vi "TitleBar.CreateBroadcasts.vi"(8 "error in (no error)":errorcluster) -> (0 "error out":errorcluster, 3 "Broadcasts":T1)   [LabVIEW 2024, in "TitleBar.lvclass"]
uses:
  TitleBar.lvclass
  Broadcast Events--cluster.ctl
  Stopped.ctl
  Maximise.ctl
  JQMHCore/Module/RQMHModule.lvclass
  Minimise.ctl
  ClosePress.ctl
  TitleBar.lvclass/TitleBar.ctl
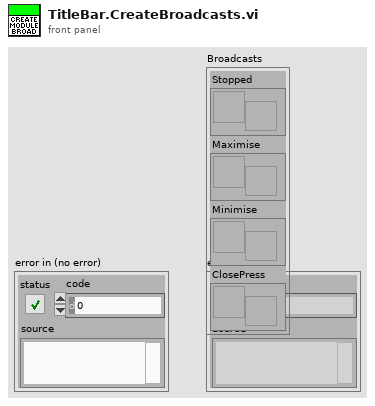
[diagram p1: front panel]
types:
  T1 = typedef "TitleBar.lvclass/Broadcast Events--cluster.ctl" = cluster{"Stopped":refnum<user-event>, "Maximise":refnum<user-event>, "Minimise":refnum<user-event>, "ClosePress":refnum<user-event>}
  T2 = typedef "TitleBar.lvclass/ClosePress.ctl" = cluster{"Module":refnum<class "RQMHModule.lvclass">}
  T3 = typedef "TitleBar.lvclass/Minimise.ctl" = cluster{"Module":refnum<class "RQMHModule.lvclass">, "null":bool}
  T4 = typedef "TitleBar.lvclass/Maximise.ctl" = cluster{"Module":refnum<class "RQMHModule.lvclass">, "Maximised":bool}
  T5 = typedef "TitleBar.lvclass/Stopped.ctl" = bool
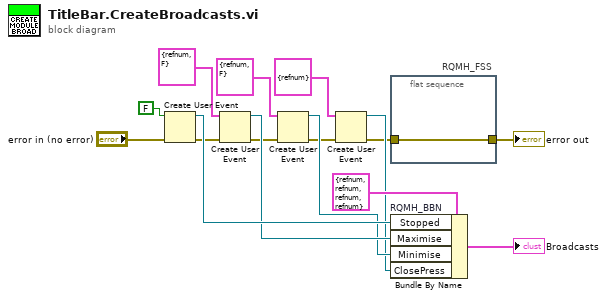
[diagram p0: block diagram]
diagram:
  n1 = Create User Event(user event datatype=T5 FALSE ("Stopped"), error in="error in (no error)") -> (user event=w15:refnum<user-event>, error out=w3:errorcluster)
  n2 = Create User Event(user event datatype=T4 {"Module"=refnum, "Maximised"=FALSE} ("Maximise"), error in=w3) -> (user event=w7:refnum<user-event>, error out=w2:errorcluster)
  n3 = Create User Event(user event datatype=T3 {"Module"=refnum, "null"=FALSE} ("Minimise"), error in=w2) -> (user event=w6:refnum<user-event>, error out=w1:errorcluster)
  n4 = Create User Event(user event datatype=T2 {"Module"=refnum} ("ClosePress"), error in=w1) -> (user event=w5:refnum<user-event>, error out=w4:errorcluster)
  n5 = flat-sequence "RQMH_FSS" {
    tunnel: w4 -> [w17]
    tunnel: [w17] -> w11
    frame #0 {
    }
  }
  n6 = Bundle By Name "RQMH_BBN"(cluster=T1 {"Stopped"=refnum, "Maximise"=refnum, "Minimise"=refnum, "ClosePress"=refnum} ("Broadcasts"), "Stopped"=w15, "Maximise"=w7, "Minimise"=w6, "ClosePress"=w5) -> (→"Broadcasts":T1)
  "error out" <- w11
